vi "Sum_Noise_Traces.vi"(9 "SumCount":u32, 10 "SumdSpectrum":dbl[](array[numeric]), 11 "AvgAvgSpectrum":dbl[](array[numeric])) -> (1 "SumCount":u32, 3 "SumdSpectrum":dbl[](array[numeric]))   [LabVIEW 2018]
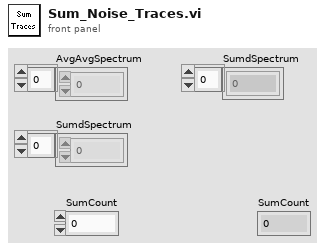
[diagram p1: front panel]
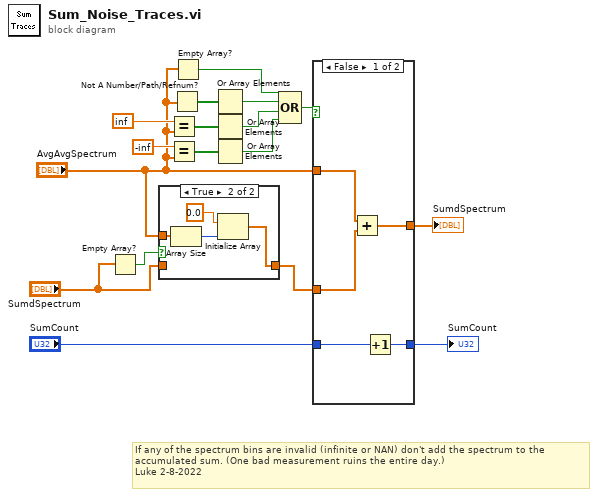
[diagram p0: block diagram]
diagram:
  # "If any of the spectrum bins are invalid (infinite or NAN) don't add the spectrum to the \naccumulated sum. (One bad measurement ruins the entire day.)\nLuke 2-8-2022"
  n1 = Empty Array?(array="SumdSpectrum") -> (empty?=w5:bool)
  n2 = case shown="True" w5 {
    tunnel: "AvgAvgSpectrum" -> [_ w22]
    tunnel: "SumdSpectrum" -> [w18 _]
    tunnel: [w18 w19] -> w3
    frame False {
    }
    frame True {
      n3 = Array Size(array=w22) -> (size(s)=w21:i32)
      n4 = Initialize Array(0.0, w21) -> (w19:dbl[])
    }
  }
  n5 = Equal?(x=inf, y="AvgAvgSpectrum") -> (x = y?=w10:bool[])
  n6 = Equal?(x=-inf, y="AvgAvgSpectrum") -> (x = y?=w11:bool[])
  n7 = Not A Number/Path/Refnum?(number/path/refnum="AvgAvgSpectrum") -> (NaN/Path/Refnum?=w12:bool[])
  n8 = Empty Array?(array="AvgAvgSpectrum") -> (empty?=w1:bool)
  n9 = Or Array Elements(Boolean array=w12) -> (logical OR=w8:bool)
  n10 = Or Array Elements(Boolean array=w10) -> (logical OR=w7:bool)
  n11 = Or Array Elements(Boolean array=w11) -> (logical OR=w6:bool)
  n12 = Compound Arithmetic op=OR(w1, w8, w7, w6) -> (w9:bool)
  n13 = case shown="False" w9 {
    tunnel: [w27 w29] -> w17
    tunnel: w3 -> [w26 w29]
    tunnel: "SumCount" -> [w25 w28]
    tunnel: [w24 w28] -> w15
    tunnel: "AvgAvgSpectrum" -> [w23 _]
    frame False {
      n14 = Add(x=w23, y=w26) -> (x+y=w27:dbl[])
      n15 = Increment(x=w25) -> (x+1=w24:u32)
    }
    frame True {
    }
  }
  "SumdSpectrum" <- w17
  "SumCount" <- w15
